vi "FFIDforceBackgroundMeas.vi"() -> ()   [LabVIEW 2014]
uses:
  Anemometry Sub Vis/Gen Trav/Traverse_cluster.ctl
  Anemometry Sub Vis/Gen Trav/Spacing.ctl
  Anemometry Sub Vis/Controls/Multi_run_mode.ctl
  Anemometry Sub Vis/Controls/User_Specific_mode.ctl
panel:
  in  "Z":dbl
  in  "Y":dbl
  in  "X":dbl
  # "Enter the location (in mm) to go to where the  background measurement is to be taken. Then run the VI, and it should take a background measurement..."
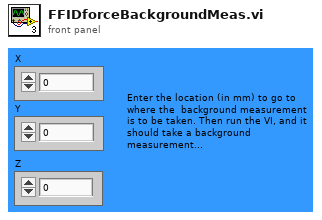
[diagram p1: front panel]
types:
  T1 = typedef "User_Specific_mode.ctl" = enum16{"Check VI only", "Run VI"}
  T2 = typedef "Traverse_cluster.ctl" = cluster{"Start X":dbl, "Start Y":dbl, "Start Z":dbl, "End X":dbl, "End Y":dbl, "End Z":dbl, "No. of pts.":i32, "Spacing":T3, "Filename":path, "Tunnel Speed":dbl, "Averaging time (min)":dbl, "Extra Commands":string, "Specific Arguments":string, "Emission Rate (l/min)":dbl, "Trace Gas Concentration (%)":dbl, "Density Ratio":string, "Comments":string, "Row No":i32, "Row Type Selector":T4, "Completion time":string, "Row Duration (mins)":dbl, "No. of Valid pts.":i32, "Meas Setup File":string}
  T3 = typedef "Spacing.ctl" = enum16{"Linear", "Log", "Gauss", "Specified", "N/A"}
  T4 = typedef "Multi_run_mode.ctl" = enum16{"Move Traverse Only", "Set Tunnel Speed Only", "Set Source Only", "Set Measurement Conditions", "Single Measurement", "Vertical Profile", "Lateral Profile", "Longitudinal Profile", "Explore Volume", "Multi-Axis Profile", "Auto Calibrate", "Meas Fast FID Bkgnd", "Check Beam Power", "Scanning Valve Measurement", "Run VI Named:", "Set ADAM Ch", "Wait (minutes)", "Send Message", "Synchronize With:", "Fall Back to this Row", "Turn Off Row Repeating", "Blank Row", "Traverse 3D Volume"}
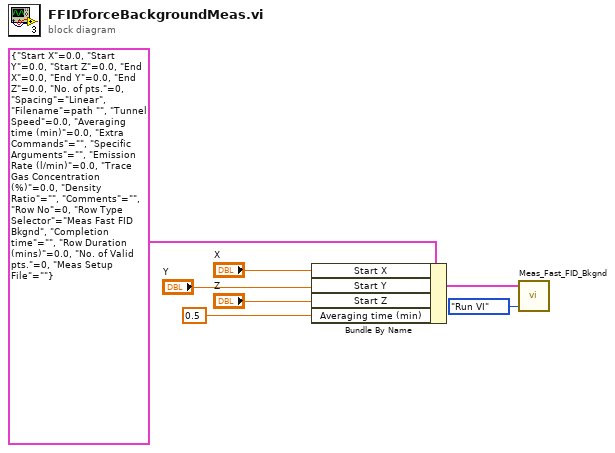
[diagram p0: block diagram]
diagram:
  n1 = Bundle By Name(cluster=T2 {"Start X"=0.0, "Start Y"=0.0, "Start Z"=0.0, "End X"=0.0, "End Y"=0.0, "End Z"=0.0, "No. of pts."=0, "Spacing"=enum."Linear", "Filename"=path "", "Tunnel Speed"=0.0, "Averaging time (min)"=0.0, "Extra Commands"="", "Specific Arguments"="", "Emission Rate (l/min)"=0.0, "Trace Gas Concentration (%)"=0.0, "Density Ratio"="", "Comments"="", "Row No"=0, "Row Type Selector"=enum."Meas Fast FID Bkgnd", "Completion time"="", "Row Duration (mins)"=0.0, "No. of Valid pts."=0, "Meas Setup File"=""} ("Traverse line In"), "Start X"="X", "Start Y"="Y", "Start Z"="Z", "Averaging time (min)"=0.5) -> (w6:T2)
  n2 = call "Meas_Fast_FID_Bkgnd.vi"("Mode"=User_Specific_mode."Run VI", "Traverse line In"=w6) -> ()  [unwired: 1 in, 3 out]
